vi "Write Commands.vi"(8 "error in (no error)":errorcluster, 10 "Commands":string[](array[string]), 11 "RemoteControl in":refnum<class "RemoteControl.lvclass">) -> (0 "error out":errorcluster, 3 "RemoteControl out":refnum<class "RemoteControl.lvclass">)   [LabVIEW 2019, in "RemoteControl.lvclass"]
uses:
  RemoteControl.lvclass
  RemoteControl.lvclass/RemoteControl.ctl
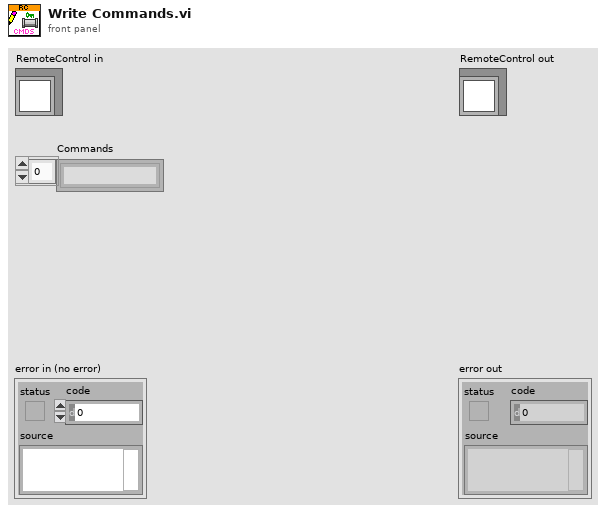
[diagram p1: front panel]
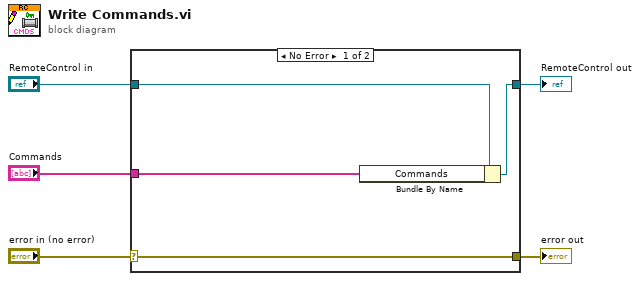
[diagram p0: block diagram]
diagram:
  n1 = case shown="No Error" "error in (no error)" {
    selector: "error in (no error)" -> [w9 w10]
    tunnel: [w9 w10] -> w4
    tunnel: [w7 w11] -> w2
    tunnel: "RemoteControl in" -> [w8 w11]
    tunnel: "Commands" -> [w6 _]
    frame No Error {
      n2 = Bundle By Name(cluster=w8, "Commands"=w6) -> (w7:refnum<class "RemoteControl.lvclass">)
    }
    frame Error {
    }
  }
  "error out" <- w4
  "RemoteControl out" <- w2
